vi "Read Positions.vi"(8 "error in (no error)":errorcluster, 11 "ArduinoFocus in":refnum<class "ArduinoFocus.lvclass">) -> (0 "error out":errorcluster, 2 "Positions":i32[](array[numeric]), 3 "ArduinoFocus out":refnum<class "ArduinoFocus.lvclass">)   [LabVIEW 2022 SP3, in "ArduinoFocus.lvclass"]
uses:
  ArduinoFocus.lvclass
  ArduinoFocus.lvclass/ArduinoFocus.ctl
  Focus Class/Focus Class.lvclass
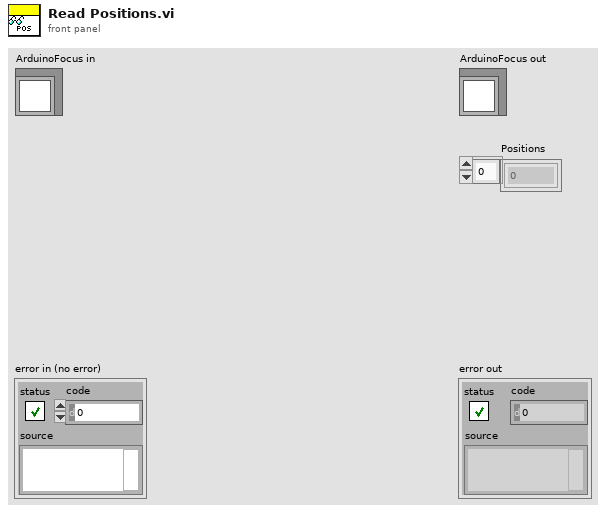
[diagram p1: front panel]
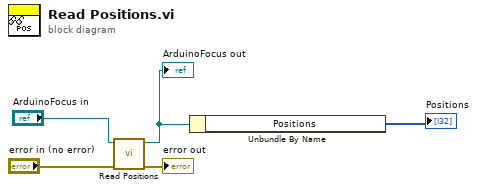
[diagram p0: block diagram]
diagram:
  n1 = call-parent "Read Positions.vi"("error in (no error)"="error in (no error)", "Focus Class in"="ArduinoFocus in") -> ("error out"=→"error out":errorcluster, "Focus Class out"=w2:refnum<class "ArduinoFocus.lvclass">)  [unwired: 7 in, 1 out]
  "ArduinoFocus out" <- w2
  n2 = Unbundle By Name(w2) -> ("Positions"=→"Positions":i32[])
